vi "485 comm RT Driver VI.vi"(6 "Device Clock":string, 9 "Device Inputs FIFO":refnum<k33>, 10 "Device Outputs FIFO":refnum<k33>, 11 "Device Reference":T1 format="%.0x") -> ()   [LabVIEW 2016, in "485 comm Custom Device.lvlib"]
uses:
  485 comm Custom Device.lvlib
  <vilib>/NI Veristand/Custom Device API/Custom Device Item Ref.ctl
  <vilib>/NI Veristand/Custom Device API/Custom Device Channel Type.ctl
  Serial - Settings.ctl
  <vilib>/NI Veristand/Custom Device API/Message Response (String).ctl
  <vilib>/NI Veristand/Custom Device API/Message Response (Byte Array).ctl
  <vilib>/NI Veristand/Custom Device API/Get Item Property (Variant).vi
  <vilib>/NI Veristand/Custom Device API/Get Item Property (String).vi
  <vilib>/Instr/_visa.llb/VISA Configure Serial Port (Instr).vi
  <vilib>/NI Veristand/Custom Device API/Custom Device API.lvlib
  <vilib>/NI Veristand/Custom Device Tools/Custom Device Utility Library/Custom Device Utility Library.lvlib
panel:
  in  "Initialization Status Notifier":refnum<notifier>
  in  "Status Notifier":refnum<notifier>
  # "Custom Device Template\nv1.0"
  # "Use this template as a starting point for creating a custom device code module. The input controls shown here are specially named controls that the system will use to provide the device loop with data. The controls are not required for the device loop to run. For instance, if the device doesn't produce any output data, then you don't need the Device Outputs FIFO control. If you do use these controls, however, they need to have these exact names to be functional."
  # "The optional status notifier element is used to notify the RT engine of the last state of the custom device, and to indicate the device has completed execution. If this control is not used, a default No Error value is returned to the system when the device finishes execution.\n\nNote: This error state is not checked until the system shuts down. Use an output status channel to send more immediate status values to the system."
  # "This optional input can be used to send the VeriStand Engine the final status of the custom device initalization process. If this control exists on the custom device front panel, the VeriStand Engine will wait for a status update before starting up. If the custom device reports an error, that will abort the execution of the current configuration in the VeriStand Engine.\n\nThis control can be deleted if the custom device does not need to send the initialization status update."
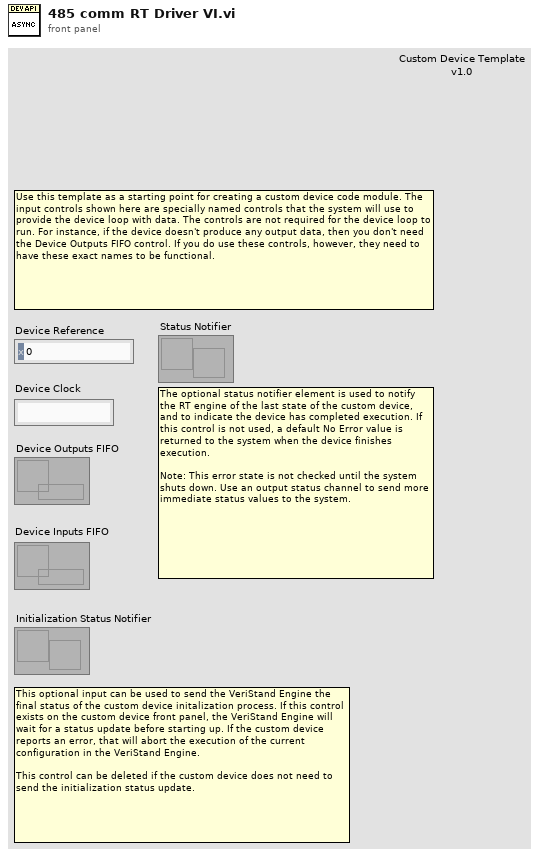
[diagram p1: front panel]
types:
  T1 = typedef "Custom Device API.lvlib/Custom Device Item Ref.ctl" = u64
  T2 = typedef "485 comm Custom Device.lvlib/Serial - Settings.ctl" = cluster{"baud rate":u32, "data bits":u16, "parity":enum16{"None", "Odd", "Even", "Mark", "Space"}, "stop bits":u16, "flow control":u16}
  T3 = typedef "Custom Device API.lvlib/Custom Device Channel Type.ctl" = enum16{"Input", "Output"}
  T4 = typedef "Custom Device API.lvlib/Custom Device Engine Event Ref.ctl" = refnum<event-registration>
  T5 = typedef "Custom Device API.lvlib/Message Response (String).ctl" = cluster{"Response":string, "Error":errorcluster}
  T6 = typedef "Custom Device API.lvlib/Message Response (Byte Array).ctl" = cluster{"Response":u8[], "Error":errorcluster}
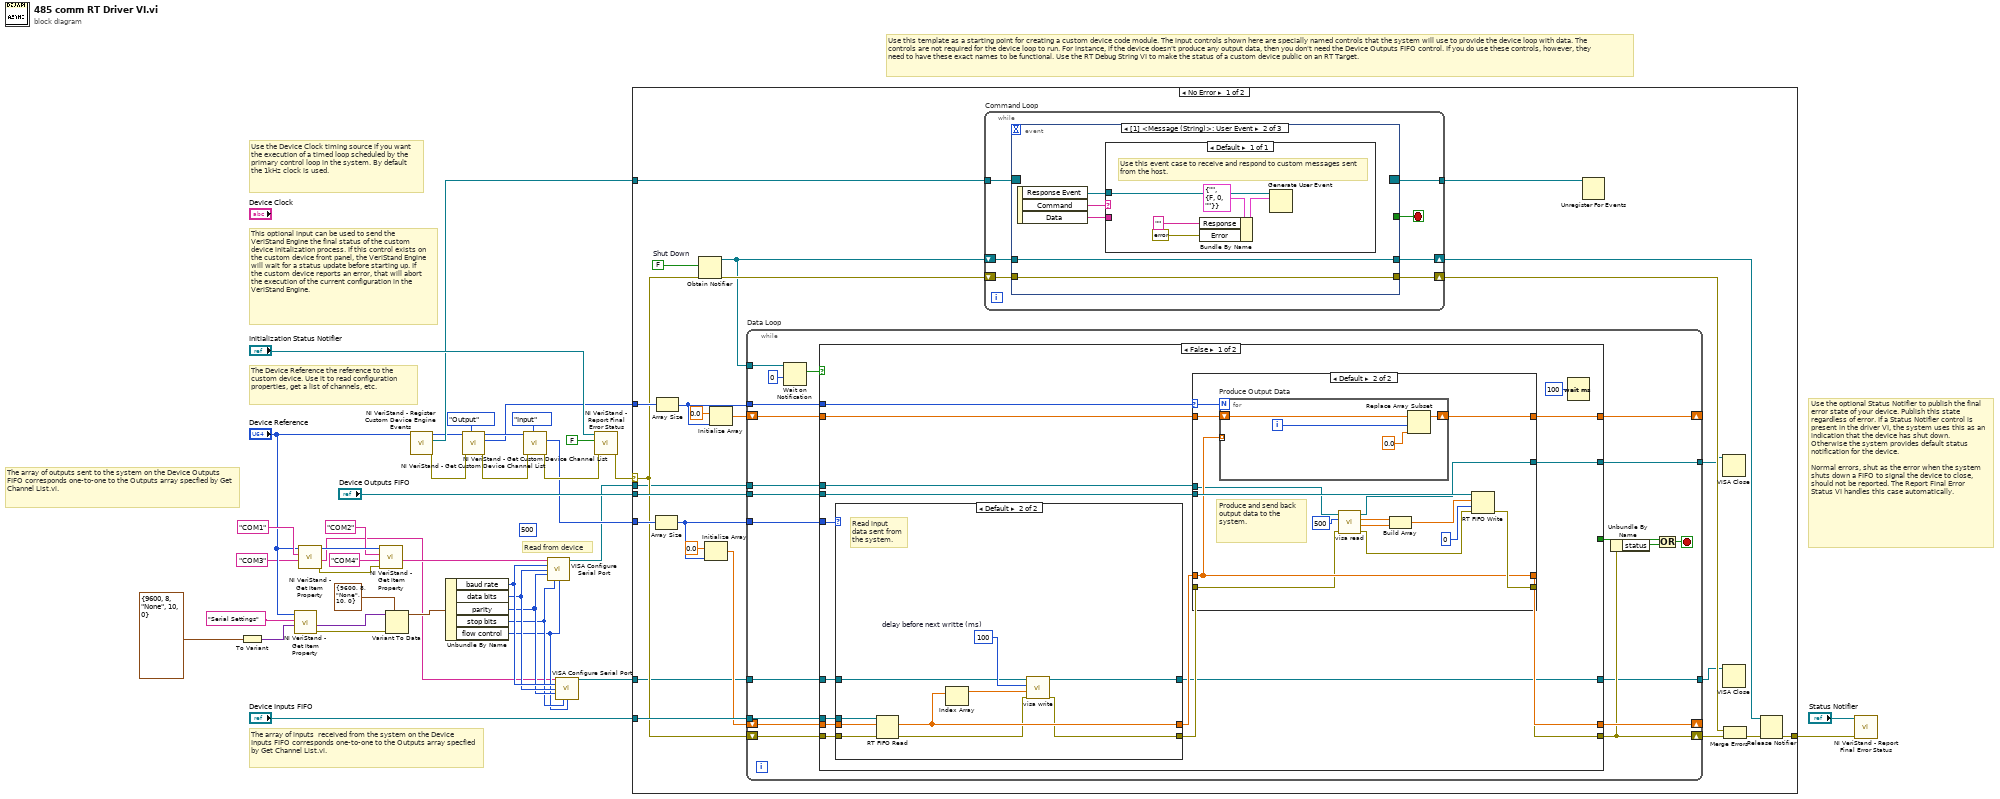
[diagram p0: block diagram]
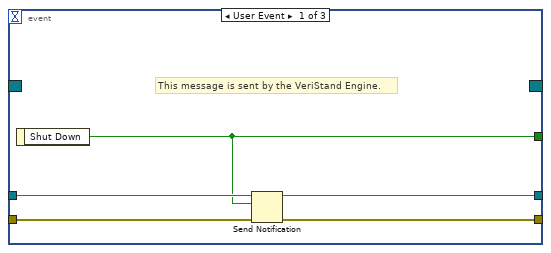
[diagram p2: hidden frame]
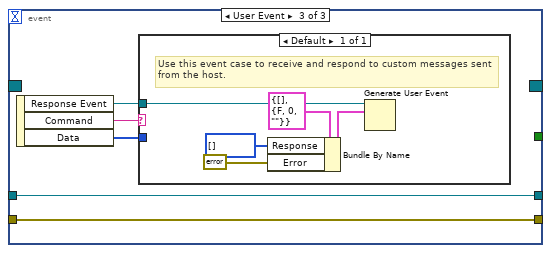
[diagram p3: hidden frame]
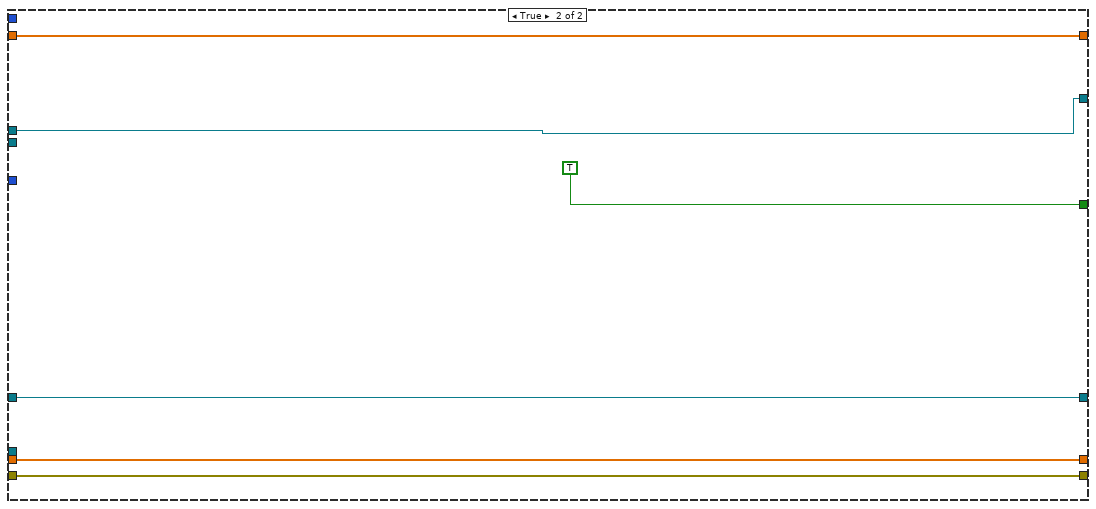
[diagram p6: hidden frame]
diagram:
  (unwired) u32 500 ("timeout (10sec)")
  # "Read from device"
  # "This optional input can be used to send the VeriStand Engine the final status of the custom device initalization process. If this control exists on the custom device front panel, the VeriStand Engine will wait for a status update before starting up. If the custom device reports an error, that will abort the execution of the current configuration in the VeriStand Engine."
  # "The array of inputs  received from the system on the Device Inputs FIFO corresponds one-to-one to the Outputs array specfied by Get Channel List.vi."
  # "Use the optional Status Notifier to publish the final error state of your device. Publish this state regardless of error. If a Status Notifier control is present in the driver VI, the system uses this as an indication that the device has shut down. Otherwise the system provides default status notification for the device.\n\nNormal errors, shut as the error when the system shuts down a FIFO to signal the device to close, should not be reported. The Report Final Error Status VI handles this case automatically."
  # "The array of outputs sent to the system on the Device Outputs FIFO corresponds one-to-one to the Outputs array specfied by Get Channel List.vi."
  # "The Device Reference the reference to the custom device. Use it to read configuration properties, get a list of channels, etc."
  # "Use the Device Clock timing source if you want the execution of a timed loop scheduled by the primary control loop in the system. By default the 1kHz clock is used."
  # "Use this template as a starting point for creating a custom device code module. The input controls shown here are specially named controls that the system will use to provide the device loop with data. The controls are not required for the device loop to run. For instance, if the device doesn't produce any output data, then you don't need the Device Outputs FIFO control. If you do use these controls, however, they need to have these exact names to be functional. Use the RT Debug String VI to make the status of a custom device public on an RT Target."
  n1 = To Variant(anything=T2 {"baud rate"=9600, "data bits"=8, "parity"=enum."None", "stop bits"=10, "flow control"=0} ("Serial Settings")) -> (Variant=w12:variant)
  n2 = call-poly <vilib>:"NI VeriStand - Get Item Property.vi"("Default Value"=w12, "Property Name"="Serial Settings", "Item Ref in"="Device Reference") -> ("error out"=w14:errorcluster, "Value"=w15:variant)  [unwired: 5 in, 2 out]
  n3 = call-poly <vilib>:"NI VeriStand - Get Item Property.vi"("Default Value"="COM3", "Property Name"="COM1", "Item Ref in"="Device Reference") -> ("error out"=w19:errorcluster, "Value"=w2:string, "Item Ref out"=w21:T1)  [unwired: 5 in, 1 out]
  n4 = call-poly <vilib>:"NI VeriStand - Get Item Property.vi"("error in (no error)"=w19, "Default Value"="COM4", "Property Name"="COM2", "Item Ref in"=w21) -> ("Value"=w10:string)  [unwired: 4 in, 3 out]
  n5 = Variant To Data(error in=w14, type=T2 {"baud rate"=9600, "data bits"=8, "parity"=enum."None", "stop bits"=10, "flow control"=0} ("Serial Settings"), Variant=w15) -> (data=w13:T2)  [unwired: 1 out]
  n6 = call <vilib>:"NI VeriStand - Register Custom Device Engine Events.vi"("Device Ref in"="Device Reference") -> ("error out"=w40:errorcluster, "Custom Device Engine Event Ref"=w28:T4, "Device Ref out"=w26:T1)  [unwired: 8 in]
  n7 = Unbundle By Name(w13) -> ("baud rate"=w7:u32, "data bits"=w6:u16, "parity"=w5:enum16{"None", "Odd", "Even", "Mark", "Space"}, "stop bits"=w4:u16, "flow control"=w3:u16)
  n8 = call <vilib>:"NI VeriStand - Get Custom Device Channel List.vi"("Channel Type"=Custom_Device_Channel_Type."Output", "error in (no error)"=w40, "Device Ref in"=w26) -> ("error out"=w33:errorcluster, "Specified Channel Ref List"=w30:T1[], "Device Ref out"=w34:T1)  [unwired: 6 out]
  n9 = call <vilib>:"NI VeriStand - Get Custom Device Channel List.vi"("Channel Type"=Custom_Device_Channel_Type."Input", "error in (no error)"=w33, "Device Ref in"=w34) -> ("error out"=w39:errorcluster, "Specified Channel Ref List"=w31:T1[])  [unwired: 7 out]
  n10 = call-poly "VISA Configure Serial Port"("VISA resource name"=w10, "baud rate (9600)"=w7, "data bits (8)"=w6, "parity (0:none)"=w5, "stop bits (10: 1 bit)"=w4, "flow control (0:none)"=w3) -> ("VISA resource name out"=w23:refnum<visa-resource-name>)  [unwired: 3 in, 6 out]
  n11 = call-poly "VISA Configure Serial Port"("VISA resource name"=w2, "baud rate (9600)"=w7, "data bits (8)"=w6, "parity (0:none)"=w5, "stop bits (10: 1 bit)"=w4, "flow control (0:none)"=w3) -> ("VISA resource name out"=w1:refnum<visa-resource-name>)  [unwired: 3 in, 6 out]
  n12 = call <vilib>:"NI VeriStand - Report Final Error Status.vi"("error in (no error)"=w39, "Filter FIFO & Shutdown Errors (T)"=FALSE ("Filter FIFO Errors (T)"), "Status Notifier"="Initialization Status Notifier") -> ("error out"=w25:errorcluster)  [unwired: 8 out]
  n13 = case shown="No Error" w25 {
    selector: w25 -> [w47 w177]
    tunnel: "Device Outputs FIFO" -> [w64 _]
    tunnel: "Device Inputs FIFO" -> [w63 _]
    tunnel: w31 -> [w57 _]
    tunnel: w30 -> [w56 _]
    tunnel: w28 -> [w54 _]
    tunnel: [w52 w177] -> w27
    tunnel: w23 -> [w44 _]
    tunnel: w1 -> [w42 _]
    frame No Error {
      w53 = FALSE  # Shut Down
      n14 = Array Size(array=w57) -> (size(s)=w55:i32)
      n15 = Array Size(array=w56) -> (size(s)=w58:i32)
      n16 = Obtain Notifier(notification data type=w53, error in (no error)=w47) -> (notifier out=w50:refnum<notifier>, error out=w65:errorcluster)  [unwired: 2 in, 1 out]
      n17 = Initialize Array(0.0 ("element"), w55) -> (w59:dbl[])
      n18 = Initialize Array(0.0 ("element"), w58) -> (w60:dbl[])
      n19 = while "Data Loop" {
        shift-right: [w115] -> _
        shift-left: w59 -> [w116]
        shift-right: [w107] -> w48
        shift-left: w47 -> [w117]
        shift-right: [w113] -> _
        shift-left: w60 -> [w114]
        tunnel: w58 -> [w110]
        tunnel: w64 -> [w112]
        tunnel: w63 -> [w111]
        tunnel: w55 -> [w109]
        tunnel: w50 -> [w106]
        tunnel: w44 -> [w101]
        tunnel: [w100] -> w43
        tunnel: w42 -> [w99]
        tunnel: [w98] -> w41
        stop <- w102 stop-if-true
        n20 = Wait on Notification(notifier=w106, timeout in ms (-1)=0) -> (notification=w105:bool)  [unwired: 2 in, 3 out]
        n21 = case shown="False" w105 {
          tunnel: w117 -> [w134 w175]
          tunnel: w116 -> [w133 w176]
          tunnel: [w132 w176] -> w115
          tunnel: w114 -> [w122 w174]
          tunnel: [w131 w174] -> w113
          tunnel: w112 -> [w130 _]
          tunnel: w111 -> [w129 _]
          tunnel: w110 -> [w128 _]
          tunnel: w109 -> [w127 _]
          tunnel: [w124 w175] -> w107
          tunnel: [_ TRUE] -> w103
          tunnel: w101 -> [w121 w172]
          tunnel: [w120 w172] -> w100
          tunnel: w99 -> [w119 w171]
          tunnel: [w118 w171] -> w98
          frame False {
            n22 = case shown="Default" w127 {
              tunnel: w129 -> [_ w170]
              tunnel: w133 -> [w160 w169]
              tunnel: [w160 w167] -> w126
              tunnel: [w159 w163] -> w125
              tunnel: w134 -> [w159 w168]
              tunnel: w119 -> [w158 w162]
              tunnel: [w158 w161] -> w118
              frame 0 {
                # "No inputs to read\nfrom system. Inputs FIFO not created in this case, so don't write to it."
              }
              frame Default {
                w165 = u32 100  # delay before next writte (ms)
                # "Read input data sent from the system."
                n23 = RT FIFO Read(0:w170, 1:w169, 3:w168) -> (9:w167:dbl[], 11:w164:errorcluster)  [unwired: 4 out]
                n24 = Index Array(array=w167) -> (element=w166:dbl)  [unwired: 1 in]
                n25 = call "visa write.vi"("error in (no error)"=w164, "input"=w166, "delay before next writte (ms)"=w165, "VISA resource name"=w162) -> ("error out"=w163:errorcluster, "VISA resource name out"=w161:refnum<visa-resource-name>)  [unwired: 6 in]
              }
            }
            n26 = case shown="Default" w128 {
              selector: w128 -> [_ w148]
              tunnel: w130 -> [_ w153]
              tunnel: w122 -> [w138 w152]
              tunnel: w126 -> [w137 w149]
              tunnel: w125 -> [w136 w139]
              tunnel: [w136 w151] -> w124
              tunnel: [w138 w150] -> w131
              tunnel: [w137 w149] -> w132
              tunnel: w121 -> [w135 w145]
              tunnel: [w135 w143] -> w120
              frame 0 {
                # "No outputs to write to system. The Device Outputs FIFO is never created in this case, so don't write to it."
              }
              frame Default {
                # "Produce and send back output data to the system."
                n27 = for "Produce Output Data" {
                  N: w148 -> [_]
                  shift-right: [w156] -> w150
                  shift-left: w152 -> [w157]
                  tunnel: w149 -> [_] mode=indexing
                  i -> [w155]
                  n28 = Replace Array Subset(array=w157, new element=0.0 ("new element/subarray"), index=w155) -> (w156:dbl[])
                }
                n29 = call "visa read.vi"("error in"=w139, "delay before read (ms)"=u32 500, "VISA resource name in"=w145) -> ("error out"=w140:errorcluster, "return count"=w142:dbl, "number"=w141:dbl, "VISA resource name out"=w143:refnum<visa-resource-name>)  [unwired: 5 in]
                n30 = Build Array(w141, w142) -> (w147:dbl[])
                n31 = RT FIFO Write(0:w153, 1:w147, 2:0 ("timeout in ms (0)"), 3:w140) -> (11:w151:errorcluster)  [unwired: 1 in, 3 out]
              }
            }
            n32 = Wait (ms)(milliseconds to wait=u32 100) -> ()  [unwired: 1 out]
          }
          frame True {
          }
        }
        n33 = Unbundle By Name(w107) -> ("status"=w104:bool)
        n34 = Compound Arithmetic op=OR(w103, w104) -> (w102:bool)
      }
      n35 = while "Command Loop" {
        tunnel: w54 -> [w72]
        tunnel: [w71] -> w51
        shift-right: [w68] -> w49
        shift-left: w50 -> [w69]
        shift-right: [w66] -> w45
        shift-left: w65 -> [w67]
        stop <- w70 stop-if-true
        n36 = event shown="[1] <Message (String)>: User Event" {
          selector: w72 -> [_ _ _]
          dyn-events: [_ _ _] -> w71
          timeout: _ -> [_ _ _]
          tunnel: [w75 _ _] -> w70
          tunnel: w69 -> [w76 w80 w90]
          tunnel: [w77 w80 w90] -> w68
          tunnel: w67 -> [w74 w78 w88]
          tunnel: [w73 w78 w88] -> w66
          event User Event {
            # "This message is sent by the VeriStand Engine."
            n37 = event-data() -> ("Shut Down"=w75:bool)  [unwired: 1 in]
            n38 = Send Notification(notification=w75, notifier=w76, error in (no error)=w74) -> (notifier out=w77:refnum<notifier>, error out=w73:errorcluster)
          }
          event User Event {
            n39 = event-data() -> ("Response Event"=w79:refnum<user-event>, "Command"=w82:string, "Data"=w81:string)  [unwired: 1 in]
            n40 = case shown="Default" w82 {
              tunnel: w81 -> [_]
              tunnel: w79 -> [w87]
              frame Default {
                # "Use this event case to receive and respond to custom messages sent from the host."
                n41 = Bundle By Name(cluster=T5 {"Response"="", "Error"={"status"=FALSE, "code"=0, "source"=""}} ("event data"), "Response"="", "Error"=errorcluster {"status"=FALSE, "code"=0, "source"=""}) -> (w85:T5)
                n42 = Generate User Event(user event=w87, event data cluster=w85) -> ()  [unwired: 2 in, 2 out]
              }
            }
          }
          event User Event {
            n43 = event-data() -> ("Response Event"=w89:refnum<user-event>, "Command"=w92:string, "Data"=w91:u8[])  [unwired: 1 in]
            n44 = case shown="Default" w92 {
              tunnel: w91 -> [_]
              tunnel: w89 -> [w97]
              frame Default {
                # "Use this event case to receive and respond to custom messages sent from the host."
                n45 = Bundle By Name(cluster=T6 {"Response"=[], "Error"={"status"=FALSE, "code"=0, "source"=""}} ("event data"), "Response"=u8[] [], "Error"=errorcluster {"status"=FALSE, "code"=0, "source"=""}) -> (w94:T6)
                n46 = Generate User Event(user event=w97, event data cluster=w94) -> ()  [unwired: 2 in, 2 out]
              }
            }
          }
        }
      }
      n47 = Unregister For Events(event registration refnum=w51) -> ()  [unwired: 1 in, 1 out]
      n48 = VISA Close(VISA resource name=w43) -> ()  [unwired: 1 in, 1 out]
      n49 = VISA Close(VISA resource name=w41) -> ()  [unwired: 1 in, 1 out]
      n50 = Merge Errors(w45, w48) -> (w46:errorcluster)
      n51 = Release Notifier(notifier=w49, error in (no error)=w46) -> (error out=w52:errorcluster)  [unwired: 1 in, 2 out]
    }
    frame Error {
    }
  }
  n52 = call <vilib>:"NI VeriStand - Report Final Error Status.vi"("error in (no error)"=w27, "Status Notifier"="Status Notifier") -> ()  [unwired: 1 in, 9 out]
